vi "DistanceFormula.vi"(10 "Point 2":cluster{"X":dbl, "Y":dbl}, 11 "Point 1":cluster{"X":dbl, "Y":dbl}) -> (3 "Distance":dbl)   [LabVIEW 2018]
doc: "Finds the distance between two points"
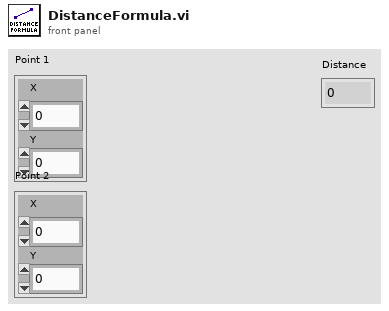
[diagram p1: front panel]
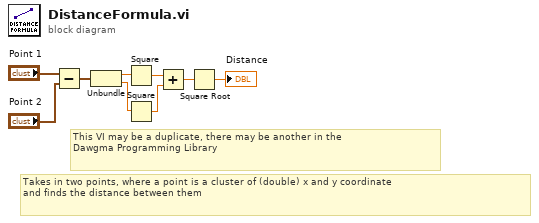
[diagram p0: block diagram]
diagram:
  # "This VI may be a duplicate, there may be another in the\nDawgma Programming Library"
  # "Takes in two points, where a point is a cluster of (double) x and y coordinate\nand finds the distance between them"
  n1 = Subtract(x="Point 1", y="Point 2") -> (x-y=w7:cluster{"X":dbl, "Y":dbl})
  n2 = Unbundle(w7) -> ("X"=w5:dbl, "Y"=w6:dbl)
  n3 = Square(x=w5) -> (x^2=w4:dbl)
  n4 = Square(x=w6) -> (x^2=w3:dbl)
  n5 = Add(x=w4, y=w3) -> (x+y=w2:dbl)
  n6 = Square Root(x=w2) -> (sqrt(x)=→"Distance":dbl)
